vi "Observe Data.vi"(6 "Time Stamp":timestamp, 8 "error in (no error)":errorcluster, 9 "Value":variant, 10 "Datum Name":string, 11 "MultiSubscriber in":refnum<class "MultiSubscriber.lvclass">) -> (0 "error out":errorcluster, 3 "MultiSubscriber out":refnum<class "MultiSubscriber.lvclass">)   [LabVIEW 2018, in "TestViewables.lvlib" / "MultiSubscriber.lvclass"]
doc: "观察数据"
uses:
  MultiSubscriber.lvclass
  modules/mva-viewable/Source/IViewable/IViewable/IViewable.lvclass
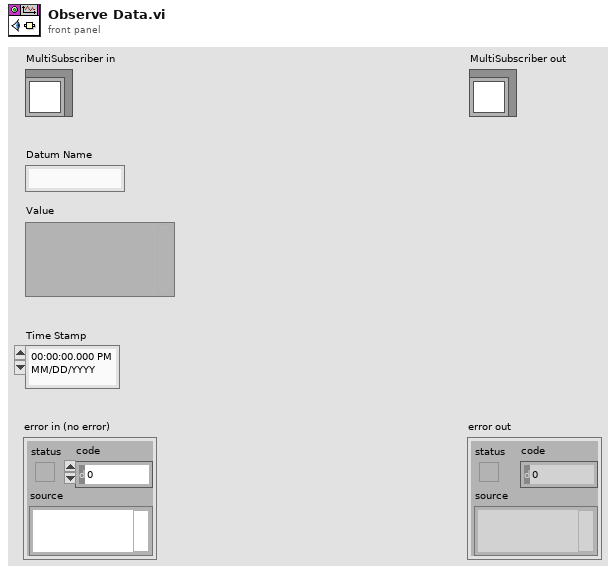
[diagram p1: front panel]
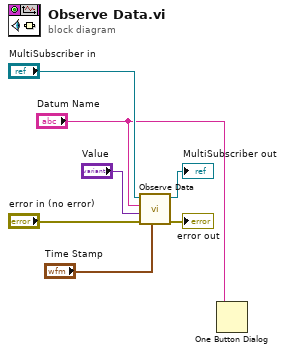
[diagram p0: block diagram]
diagram:
  n1 = call-parent "Observe Data.vi"("Time Stamp"="Time Stamp", "error in (no error)"="error in (no error)", "Value"="Value", "Datum Name"="Datum Name", "IObserver in"="MultiSubscriber in") -> ("error out"=→"error out":errorcluster, "IObserver out"=→"MultiSubscriber out":refnum<class "MultiSubscriber.lvclass">)  [unwired: 5 in]
  n2 = One Button Dialog(message="Datum Name") -> ()  [unwired: 1 in, 1 out]
